vi "test Get and Set Engine Pointer.vi"(8 "error in (no error)":errorcluster, 11 "TestCase in":refnum<class "Framework Tests.lvclass">) -> (0 "error out":errorcluster, 3 "TestCase out":refnum<class "Framework Tests.lvclass">)   [LabVIEW 2017, in "Framework Tests.lvclass"]
uses:
  Framework Tests.lvclass
  Mock Framework Class/Mock Framework.lvclass
  C:/github/data-sharing-framework/Data Sharing Framework Core/Engine/Classes/Framework/Framework.lvclass
  <vilib>/NI/Memory Manager/Classes/Pointer/Pointer.lvclass/Pointer.ctl
  Engine/Classes/Framework/Framework.lvclass/Framework.ctl
  <vilib>/NI/Memory Manager/Classes/Pointer/Public/New/New (1B).vi
  <vilib>/NI/Memory Manager/Classes/Pointer/Private/Allocate.vi
  <vilib>/NI/Memory Manager/Classes/Pointer/API/Accessors/Set Address.vi
  <vilib>/NI/Memory Manager/Classes/Pointer/API/Accessors/Set Size.vi
  <vilib>/NI/Memory Manager/Classes/Pointer/Private/Set Internal.vi
  <vilib>/NI/Memory Manager/Classes/Pointer/Pointer.lvclass
  <vilib>/addons/_JKI Toolkits/VI Tester/TestCase.llb/TestCase.lvclass
  Engine/Classes/Framework/Framework.lvclass
  C:/Program Files (x86)/National Instruments/LabVIEW 2017/vi.lib/addons/_JKI Toolkits/VI Tester/TestCase.llb/TestCase.lvclass
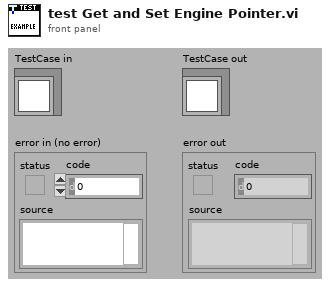
[diagram p1: front panel]
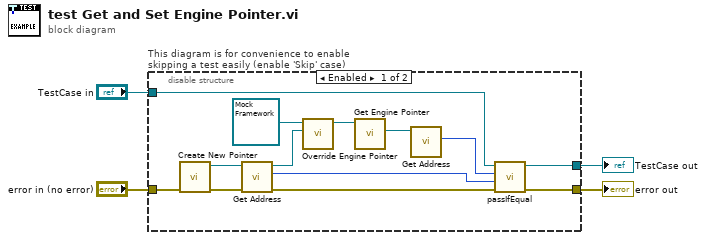
[diagram p0: block diagram]
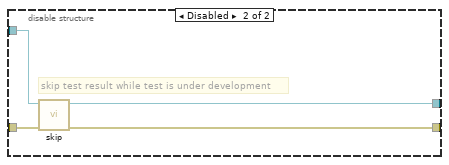
[diagram p2: hidden frame]
diagram:
  n1 = disable-structure "This diagram is for convenience to enable skipping a test easily (enable 'Skip' case)" shown="Enabled" {
    disable-tunnel: "TestCase in" -> [w15 w20]
    disable-tunnel: [w14 w18] -> w2
    disable-tunnel: [w16 w19] -> w1
    disable-tunnel: "error in (no error)" -> [w10 w17]
    frame Enabled {
      n2 = call-poly <vilib>:"Create New Pointer.vi"("error in (no error)"=w10) -> ("error out"=w9:errorcluster, "Pointer"=w11:refnum<class "Pointer.lvclass">)  [unwired: 9 in]
      n3 = call <vilib>:"Get Address.vi"("Pointer in"=w11) -> ("address"=w7:u64, "Pointer out"=w8:refnum<class "Pointer.lvclass">)  [unwired: 9 in]
      n4 = call "Override Engine Pointer.vi"("Engine Pointer"=w8, "Mock Framework in"=refnum<class "Mock Framework.lvclass"> refnum) -> ("Mock Framework out"=w13:refnum<class "Mock Framework.lvclass">)  [unwired: 8 in, 1 out]
      n5 = call "Get Engine Pointer.vi"("Framework in"=w13) -> ("Engine Pointer"=w6:refnum<class "Pointer.lvclass">)  [unwired: 9 in, 1 out]
      n6 = call <vilib>:"Get Address.vi"("Pointer in"=w6) -> ("address"=w5:u64)  [unwired: 9 in, 1 out]
      n7 = call-dynamic "passIfEqual.vi"("error in (no error)"=w9, "y"=w7, "x"=w5, "TestCase in"=w15) -> ("error out"=w16:errorcluster, "TestCase out"=w14:refnum<class "Framework Tests.lvclass">)  [unwired: 6 in]
    }
    frame Disabled {
      # "skip test result while test is under development"
      n8 = call <vilib>:"skip.vi"("error in (no error)"=w17, "TestCase in"=w20) -> ("error out"=w19:errorcluster, "TestCase out"=w18:refnum<class "Framework Tests.lvclass">)  [unwired: 8 in]
    }
  }
  "error out" <- w1
  "TestCase out" <- w2
